vi "Text as Encoded String (LabVIEW String).vi"(6 "error in":errorcluster, 9 "Text":string) -> (1 "Encoded String":T1, 4 "error out":errorcluster)   [LabVIEW 2020, in "G-Unicode.lvlib"]
doc: "Converts the input string or path to a raw UTF-8 encoded LabVIEW string. Valid inputs are a UTF-8 String class, UTF-8 Path class, LabVIEW string, or LabVIEW path."
uses:
  Types/UTF-8 String/UTF-8 String.lvclass/UTF-8 String.ctl
  G-Unicode.lvlib
  Types/Encoded UTF-8 String.ctl
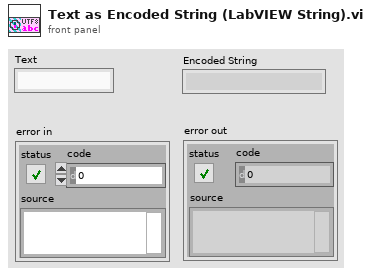
[diagram p1: front panel]
types:
  T1 = typedef "G-Unicode.lvlib/Encoded UTF-8 String.ctl" = string
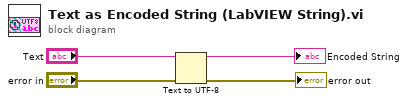
[diagram p0: block diagram]
diagram:
  n1 = Text to UTF-8(8:"error in", 11:"Text") -> (0:→"error out":errorcluster, 3:→"Encoded String":string)  [unwired: 1 in]
